vi "Sweeping Turn.vi"(5 "PID gains":T1={"proportional gain (Kc)"=1.0, "integral time (Ti, min)"=0.01, "derivative time (Td, min)"=0.0} {"derivative time (Td, min)" format="%.3f"; "integral time (Ti, min)" format="%.3f"; "proportional gain (Kc)" format="%.3f"}, 6 "Target Yaw":dbl, 8 "error in":errorcluster, 9 "Acceptable Range":dbl) -> (0 "error out":errorcluster, 2 "Yaw":dbl, 3 "Yaw Output":dbl format="%.2f", 4 "Stop":bool)   [LabVIEW 2017]
uses:
  <vilib>/addons/control/pid/pid.llb/PID (DBL).vi
  <vilib>/addons/control/pid/NI_PID_pid.lvlib
panel:
  out "Target Yaw out":dbl
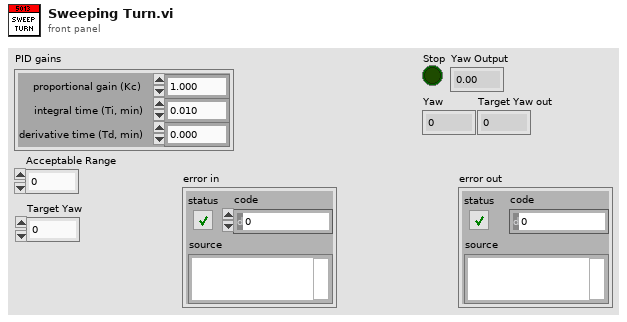
[diagram p1: front panel]
types:
  T1 = cluster{"proportional gain (Kc)":dbl, "integral time (Ti, min)":dbl, "derivative time (Td, min)":dbl}
  T2 = cluster{"Yaw":dbl, "Roll":dbl, "Pitch":dbl, "Heading":dbl, "Fused Heading":dbl}
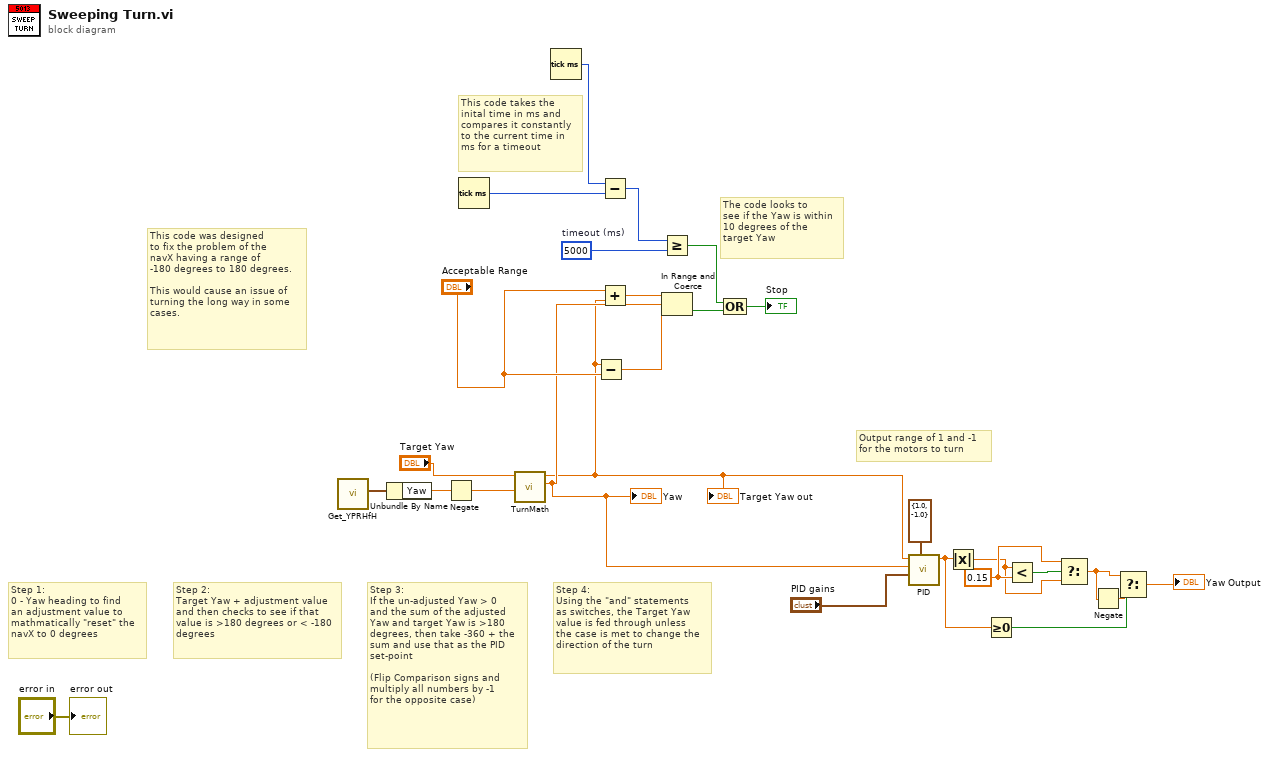
[diagram p0: block diagram]
diagram:
  w7 = 0.15 ("y")
  w19 = u32 5000  # timeout (ms)
  # "This code was designed\nto fix the problem of the\nnavX having a range of \n-180 degrees to 180 degrees.\n\nThis would cause an issue of\nturning the long way in some\ncases."
  # "Output range of 1 and -1\nfor the motors to turn"
  # "Step 4:\nUsing the \"and\" statements\nas switches, the Target Yaw\nvalue is fed through unless\nthe case is met to change the\ndirection of the turn"
  # "Step 3:\nIf the un-adjusted Yaw > 0 \nand the sum of the adjusted \nYaw and target Yaw is >180\ndegrees, then take -360 + the \nsum and use that as the PID \nset-point\n\n(Flip Comparison signs and\nmultiply all numbers by -1 \nfor the opposite case)"
  # "Step 2:\nTarget Yaw + adjustment value\nand then checks to see if that \nvalue is >180 degrees or < -180\ndegrees"
  # "Step 1: \n0 - Yaw heading to find\nan adjustment value to \nmathmatically \"reset\" the\nnavX to 0 degrees"
  # "The code looks to \nsee if the Yaw is within\n10 degrees of the \ntarget Yaw"
  # "This code takes the\ninital time in ms and\ncompares it constantly\nto the current time in\nms for a timeout"
  n1 = call <vilib>:"Get_YPRHfH.vi"() -> ("YRPHfH"=w13:T2)  [unwired: 11 in]
  n2 = Unbundle By Name(w13) -> ("Yaw"=w12:dbl)
  n3 = Negate(x=w12) -> (-x=w11:dbl)
  n4 = Tick Count (ms)() -> (millisecond timer value=w26:u32)
  n5 = call "TurnMath.vi"("Yaw in"=w11, "Target Yaw in"="Target Yaw") -> ("Yaw out"=w10:dbl, "Target Yaw out"=w9:dbl)  [unwired: 8 in]
  "Yaw" <- w10
  "Target Yaw out" <- w9
  n6 = Tick Count (ms)() -> (millisecond timer value=w23:u32)
  n7 = Subtract(x=w9, y="Acceptable Range") -> (x-y=w17:dbl)
  n8 = Subtract(x=w23, y=w26) -> (x-y=w22:u32)
  n9 = Add(x="Acceptable Range", y=w9) -> (x+y=w16:dbl)
  n10 = Greater Or Equal?(x=w22, y=w19) -> (x >= y?=w20:bool)
  n11 = In Range and Coerce(upper limit=w16, x=w10, lower limit=w17) -> (In Range?=w18:bool)  [unwired: 1 out]
  n12 = Compound Arithmetic op=OR(w20, w18) -> (→"Stop":bool)
  n13 = call-poly <vilib>:"PID.vi"("output range"=cluster{"output high":dbl, "output low":dbl} {"output high"=1.0, "output low"=-1.0}, "PID gains"="PID gains", "process variable"=w10, "setpoint"=w9) -> ("output"=w5:dbl)  [unwired: 6 in, 1 out]
  n14 = Absolute Value(x=w5) -> (abs(x)=w6:dbl)
  n15 = Greater Or Equal To 0?(x=w5) -> (x >= 0?=w4:bool)
  n16 = Less?(x=w6, y=w7) -> (x < y?=w8:bool)
  n17 = Select(t=w7, s=w8, f=w6) -> (s? t:f=w2:dbl)
  n18 = Negate(x=w2) -> (-x=w3:dbl)
  n19 = Select(t=w2, s=w4, f=w3) -> (s? t:f=→"Yaw Output":dbl)
  "error out" <- "error in"
